vi "Convert Counts per Interval to Radians per Second.vi"(10 "interval (ticks)":fxp<+,23,23>=320000.0, 11 "velocity (pulses/interval)":fxp<+/-,6,6>) -> (3 "velocity (rad/s)":fxp<+/-,32,11> format="%.39g")   [LabVIEW 2011]
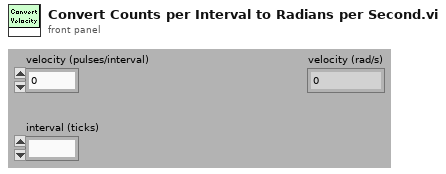
[diagram p1: front panel]
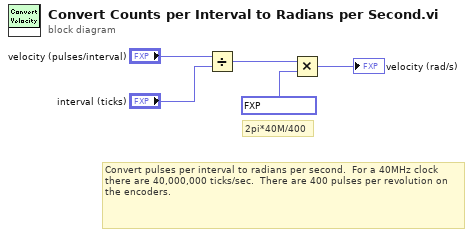
[diagram p0: block diagram]
diagram:
  # "Convert pulses per interval to radians per second.  For a 40MHz clock there are 40,000,000 ticks/sec.  There are 400 pulses per revolution on the encoders."
  # "2pi*40M/400"
  n1 = Divide(x="velocity (pulses/interval)", y="interval (ticks)") -> (x/y=w3:fxp<+/-,32,1>)
  n2 = Multiply(x=w3, y=fxp<+,31,22> 628318.53125) -> (x*y=→"velocity (rad/s)":fxp<+/-,32,11>)
